vi "Copy.vi"(0 "Tree Data":refnum<class "Tree Data.lvclass">, 11 "Error In":errorcluster) -> (4 "Original":refnum<class "Tree Data.lvclass">, 6 "Copy":refnum<class "Tree Data.lvclass">, 15 "Error Out":errorcluster)   [LabVIEW 2016, in "Tree Data.lvclass"]
uses:
  Tree Data.lvclass
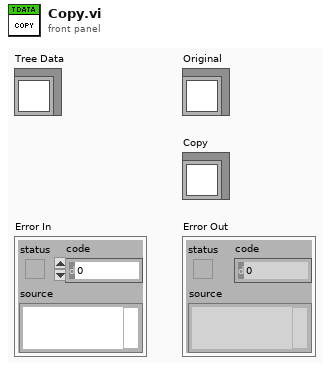
[diagram p1: front panel]
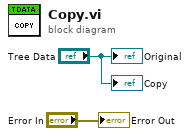
[diagram p0: block diagram]
diagram:
  "Error Out" <- "Error In"
  "Original" <- "Tree Data"
  "Copy" <- "Tree Data"
